vi "Table, Copy Column Headers.vi"(4 "error in":errorcluster, 6 "Tbl Refnum Dst":refnum<vi>, 7 "Tbl Refnum Src":refnum<vi>) -> (0 "error out":errorcluster, 2 "Tbl Refnum Dst out":refnum<vi>, 3 "Tbl Refnum Src out":refnum<vi>)   [LabVIEW 2010]
doc: "Copies the column headers (labels) of the source table to the destination table."
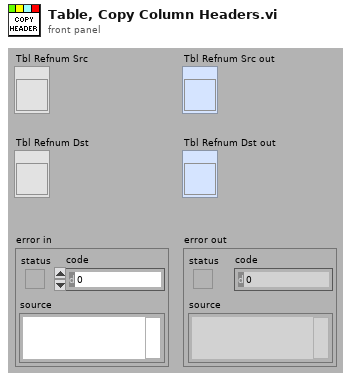
[diagram p1: front panel]
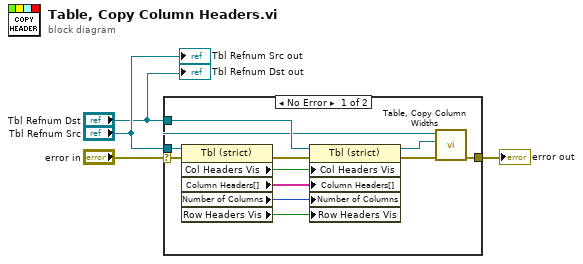
[diagram p0: block diagram]
diagram:
  n1 = case shown="No Error" "error in" {
    selector: "error in" -> [w5 w16]
    tunnel: [w10 w16] -> w4
    tunnel: "Tbl Refnum Dst" -> [w7 _]
    tunnel: "Tbl Refnum Src" -> [w6 _]
    frame No Error {
      n2 = property class="Tbl (strict)"(reference=w6, error in=w5) -> (error out=w13:errorcluster, "Col Headers Vis"=w15:bool, "Column Headers[]"=w14:string[], "Number of Columns"=w12:u32, "Row Headers Vis"=w8:bool)  [unwired: 1 out]
      n3 = property class="Tbl (strict)"(reference=w7, error in=w13, "Col Headers Vis"=w15, "Column Headers[]"=w14, "Number of Columns"=w12, "Row Headers Vis"=w8) -> (reference out=w9:refnum<vi>, error out=w11:errorcluster)
      n4 = call "Table, Copy Column Widths.vi"("error in"=w11, "Tbl Refnum Dst"=w9, "Tbl Refnum Src"=w6) -> ("error out"=w10:errorcluster)  [unwired: 2 in, 2 out]
    }
    frame Error {
    }
  }
  "error out" <- w4
  "Tbl Refnum Src out" <- "Tbl Refnum Src"
  "Tbl Refnum Dst out" <- "Tbl Refnum Dst"
